vi "Set DDG External Output Time.vi"(9 "uiWidth":cluster{}, 10 "uiDelay":cluster{}, 11 "uiIndex":u32) -> (3 "function return":u32)   [LabVIEW 2018, in "AndorSDK.lvlib"]
doc: "EXPNETTYPE unsigned int WINAPI SetDDGExternalOutputTime(at_u32 uiIndex, at_u64 uiDelay, at_u64 uiWidth);"
uses:
  AndorSDK.lvlib
  ATMCD32D.dll
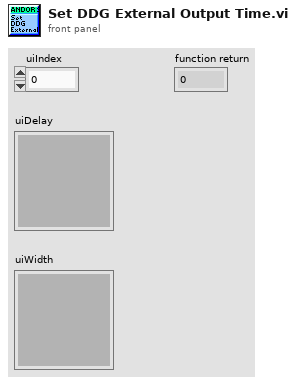
[diagram p1: front panel]
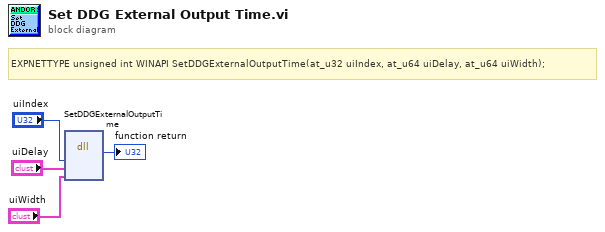
[diagram p0: block diagram]
diagram:
  # "EXPNETTYPE unsigned int WINAPI SetDDGExternalOutputTime(at_u32 uiIndex, at_u64 uiDelay, at_u64 uiWidth);"
  n1 = dll-call lib="PTH2babs E\nPersönliches02 - Arbeit03-HiwijobsLabviewCodelibANDOR\tAndor SDK\nATMCD32D.*" fn="SetDDGExternalOutputTime"("uiIndex"="uiIndex", "uiDelay"="uiDelay", "uiWidth"="uiWidth") -> (→"function return":u32)  [unwired: 6 in, 2 out]
